vi "Calculate INL.vi"(0 "Actual X":dbl[](array[numeric]), 1 "Best Fit?":bool, 5 "Actual Y":dbl[](array[numeric]), 7 "Ideal X":dbl[](array[numeric]), 9 "Ideal Y":dbl[](array[numeric]), 11 "Error in":errorcluster, 12 "ADC?":bool) -> (4 "INL Y Plot Values":dbl[](array[numeric]), 8 "INL Result values":dbl[](array[numeric]), 15 "Error out":errorcluster)   [LabVIEW 2020, in "INL DNL Test.lvclass"]
doc: "Calculates INL result based on bestfit/endpoint method"
uses:
  INL DNL Test.lvclass
  <vilib>/Analysis/6fits.llb/Curve Fitting Criteria.ctl
  <vilib>/Analysis/NI_AALPro.lvlib
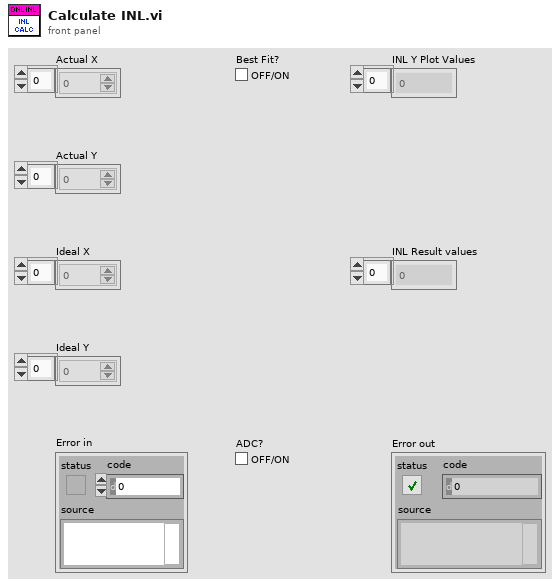
[diagram p1: front panel]
types:
  T1 = typedef "NI_AALPro.lvlib/Curve Fitting Criteria.ctl" = u16
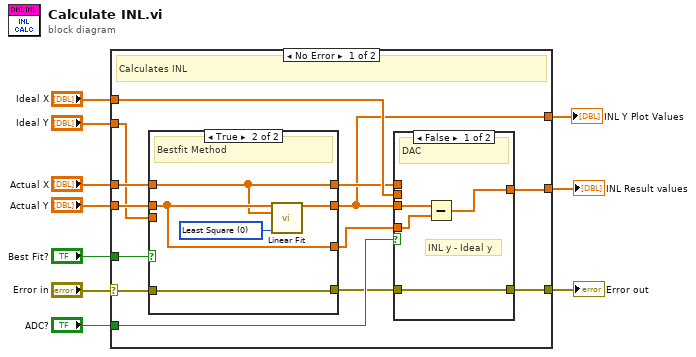
[diagram p0: block diagram]
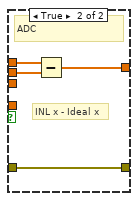
[diagram p3: hidden frame]
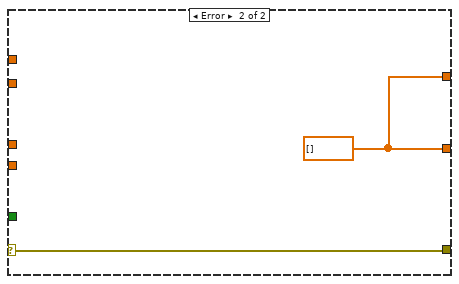
[diagram p4: hidden frame]
diagram:
  n1 = case shown="No Error" "Error in" {
    selector: "Error in" -> [w20 w42]
    tunnel: "Best Fit?" -> [w23 _]
    tunnel: "Actual X" -> [w22 _]
    tunnel: "Actual Y" -> [w21 _]
    tunnel: "Ideal X" -> [w18 _]
    tunnel: "Ideal Y" -> [w12 _]
    tunnel: "ADC?" -> [w19 _]
    tunnel: [w15 w42] -> w2
    tunnel: [w14 w41] -> w3
    tunnel: [w11 w41] -> w1
    frame No Error {
      # "Calculates INL"
      n2 = case shown="True" w23 {
        tunnel: w22 -> [w27 w28]
        tunnel: w21 -> [w25 w29]
        tunnel: [w25 w31] -> w11
        tunnel: [w27 w28] -> w17
        tunnel: w20 -> [w26 w30]
        tunnel: [w26 w30] -> w16
        tunnel: [w24 w29] -> w13
        tunnel: w12 -> [w24 _]
        frame False {
          # "Endpoint Method"
        }
        frame True {
          w32 = T1 0 items=["Least Square", "Least Absolute Residual", "Bisquare"] ("method")
          # "Bestfit Method"
          n3 = call <vilib>:"Linear Fit.vi"("Y"=w29, "X"=w28, "method"=w32) -> ("Best Linear Fit"=w31:dbl[])  [unwired: 8 in, 4 out]
        }
      }
      n4 = case shown="False" w19 {
        tunnel: w18 -> [_ w38]
        tunnel: w17 -> [_ w39]
        tunnel: [w35 w40] -> w14
        tunnel: w11 -> [w36 _]
        tunnel: w16 -> [w34 w37]
        tunnel: [w34 w37] -> w15
        tunnel: w13 -> [w33 _]
        frame False {
          # "INL y - Ideal y"
          # "DAC"
          n5 = Subtract(x=w36, y=w33) -> (x-y=w35:dbl[])
        }
        frame True {
          # "INL x - Ideal x"
          # "ADC"
          n6 = Subtract(x=w39, y=w38) -> (x-y=w40:dbl[])
        }
      }
    }
    frame Error {
      w41 = dbl[] []
    }
  }
  "INL Result values" <- w3
  "Error out" <- w2
  "INL Y Plot Values" <- w1
